vi "Update Listbox.vi"(9 "Mandatory":string[](array[string]), 10 "Data In":T1, 11 "ListBox in":refnum<vi>) -> (0 "error out":errorcluster, 3 "ListBox out":refnum<vi>)   [LabVIEW 2015, in "Editable I-O Listbox.xctl"]
uses:
  Editable I-O Listbox.xctl
  Data.ctl
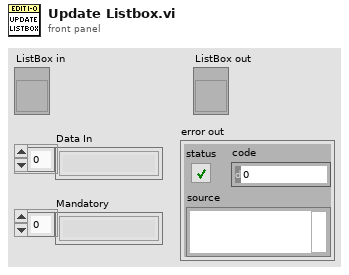
[diagram p1: front panel]
types:
  T1 = typedef "Editable I-O Listbox.xctl/Data.ctl" = string[]
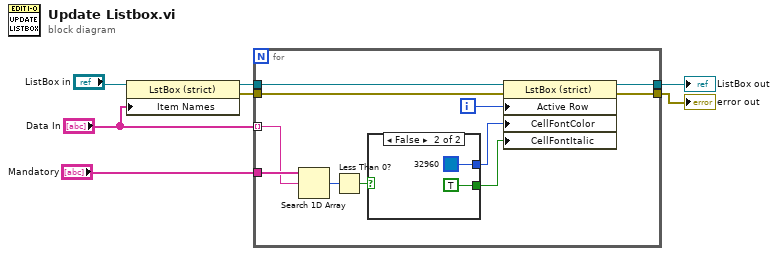
[diagram p0: block diagram]
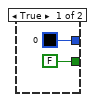
[diagram p2: hidden frame]
diagram:
  n1 = property class="LstBox (strict)"(reference="ListBox in", "Item Names"="Data In") -> (reference out=w5:refnum<vi>, error out=w3:errorcluster)  [unwired: 1 in]
  n2 = for {
    tunnel: "Data In" -> [w17] mode=indexing
    tunnel: "Mandatory" -> [w18]
    tunnel: w5 -> [w16]
    tunnel: w3 -> [w15]
    tunnel: [w9] -> w2
    tunnel: [w8] -> w1
    i -> [w14]
    n3 = Search 1D Array(1D array=w18, element=w17) -> (index of element=w13:i32)  [unwired: 1 in]
    n4 = Less Than 0?(x=w13) -> (x < 0?=w12:bool)
    n5 = case shown="False" w12 {
      tunnel: [u32 0 u32 32960] -> w11
      tunnel: [FALSE TRUE] -> w10
      frame True {
      }
      frame False {
      }
    }
    n6 = property class="LstBox (strict)"(reference=w16, error in=w15, "Active Row"=w14, "CellFontColor"=w11, "CellFontItalic"=w10) -> (reference out=w9:refnum<vi>, error out=w8:errorcluster)
  }
  "ListBox out" <- w2
  "error out" <- w1
